vi "PC_Find_Reference_Dot (DONE).vi"(7 "Number of Erosion in":i32, 8 "Error In":errorcluster, 11 "Image In":T1) -> (0 "Error Out":errorcluster, 2 "Reference Dimentions Out":cluster{"X":dbl, "Y":dbl, "Width":dbl}, 3 "Image Out":T1)   [LabVIEW 2017]
uses:
  <vilib>/vision/Image Controls.llb/IMAQ Image.ctl
  <vilib>/vision/NI_Vision_Development_Module.lvlib
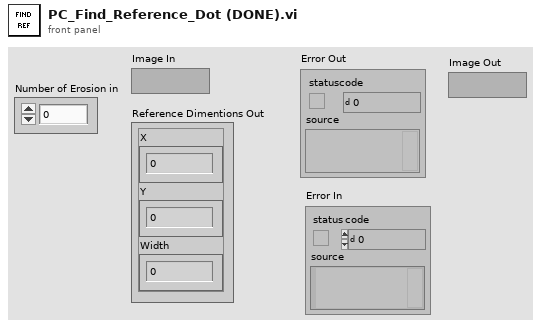
[diagram p1: front panel]
types:
  T1 = typedef "IMAQ Image.ctl" = refnum<image>
  T2 = typedef "ROI Descriptor" = cluster{"Global Rectangle":i32[], "Contours":cluster{"ID":enum32{"External", "Internal"}, "Type":u32, "Coordinates":i32[]}[]}
  T3 = cluster{"Area":dbl, "Number of Holes":dbl, "Bounding Rect":cluster{"Left":dbl, "Top":dbl, "Right":dbl, "Bottom":dbl}, "Center of Mass":cluster{"X":dbl, "Y":dbl}, "Orientation":dbl, "Dimensions":cluster{"Width":dbl, "Height":dbl}}[]
  T4 = cluster{"Area":dbl, "Number of Holes":dbl, "Bounding Rect":cluster{"Left":dbl, "Top":dbl, "Right":dbl, "Bottom":dbl}, "Center of Mass":cluster{"X":dbl, "Y":dbl}, "Orientation":dbl, "Dimensions":cluster{"Width":dbl, "Height":dbl}}
  T5 = cluster{"Left":dbl, "Top":dbl, "Right":dbl, "Bottom":dbl}
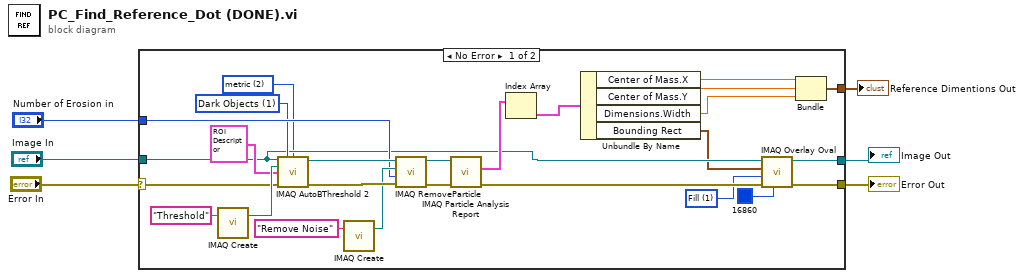
[diagram p0: block diagram]
diagram:
  n1 = case shown="No Error" "Error In" {
    selector: "Error In" -> [w23 w34]
    tunnel: "Number of Erosion in" -> [w29 _]
    tunnel: [w17 w34] -> w5
    tunnel: [w15 w33] -> w4
    tunnel: "Image In" -> [w16 w33]
    tunnel: [w9 _] -> w1
    frame No Error {
      w7 = 2 items=["clustering", "entropy", "metric", "moments", "inter-class variance"] ("Method (clustering)")
      w13 = u32 1 items=["Frame", "Fill"] ("Drawing Mode (Frame)")
      w25 = u32 1 items=["Bright Objects", "Dark Objects"] ("Look For (Bright Objects)")
      n2 = call "IMAQ Create"("Image Name"="Threshold") -> ("New Image"=w28:T1)  [unwired: 4 in, 1 out]
      n3 = call "IMAQ AutoBThreshold 2"("Image Src"=w16, "Look For (Bright Objects)"=w25, "Method (clustering)"=w7, "Image Dst"=w28, "ROI Descriptor"=T2 {"Global Rectangle"=[649, 354, 965, 688], "Contours"=[{"ID"=enum."External", "Type"=12, "Coordinates"=[649, 354, 965, 688, 0]}]}, "error in (no error)"=w23) -> ("Image Dst Out"=w32:T1, "error out"=w31:errorcluster)  [unwired: 7 in, 1 out]
      n4 = call "IMAQ Create"("Image Name"="Remove Noise") -> ("New Image"=w30:T1)  [unwired: 4 in, 1 out]
      n5 = call "IMAQ RemoveParticle"("error in (no error)"=w31, "Number of Erosion"=w29, "Image Dst"=w30, "Image Src"=w32) -> ("error out"=w22:errorcluster, "Image Dst Out"=w21:T1)  [unwired: 6 in]
      n6 = call "IMAQ Particle Analysis Report"("error in (no error)"=w22, "Image"=w21) -> ("error out"=w20:errorcluster, "Particle Reports (Pixels)"=w19:T3)  [unwired: 4 in, 4 out]
      n7 = Index Array(array=w19) -> (element=w18:T4)  [unwired: 1 in]
      n8 = Unbundle By Name(w18) -> ("Center of Mass.X"=w12:dbl, "Center of Mass.Y"=w11:dbl, "Dimensions.Width"=w10:dbl, "Bounding Rect"=w8:T5)
      n9 = call "IMAQ Overlay Oval"("Color"=u32 16860, "error in (no error)"=w20, "Drawing Mode (Frame)"=w13, "Bounding Rectangle"=w8, "Image"=w16) -> ("error out"=w17:errorcluster, "Image Out"=w15:T1)  [unwired: 5 in]
      n10 = Bundle("X"=w12, "Y"=w11, "Width"=w10) -> (w9:cluster{"X":dbl, "Y":dbl, "Width":dbl})  [unwired: 1 in]
    }
    frame Error {
    }
  }
  "Error Out" <- w5
  "Image Out" <- w4
  "Reference Dimentions Out" <- w1
